vi "Configure Integration.vi"(8 "error in (no error)":errorcluster, 10 "Integration Time (5: 1PLC)":i32(ring)=5 items=["100us", "500us", "1ms", "5ms", "10ms", "1PLC", "100ms", "200ms", "Sample Hold(100 ms)"], 11 "VISA resource name":refnum<visa-resource-name>) -> (0 "error out":errorcluster, 3 "VISA resource name out":refnum<visa-resource-name>)   [LabVIEW 2017, in "ADCMT 6240.lvlib"]
doc: "This VI configures the integration time on the instrument.\n\n<B>Note:</B> Sample Hold can set only at the pulse mode, the pulse-RM mode or the pulse sweep mode."
uses:
  ADCMT 6240.lvlib
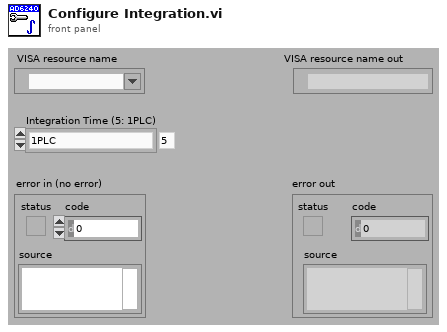
[diagram p1: front panel]
types:
  T1 = typedef "ADCMT 6240.lvlib/Extended User Data.ctl" = cluster{"Trigger Mode":u16, "Output Mode":u16, "Sample Count":i32, "Model":u16}
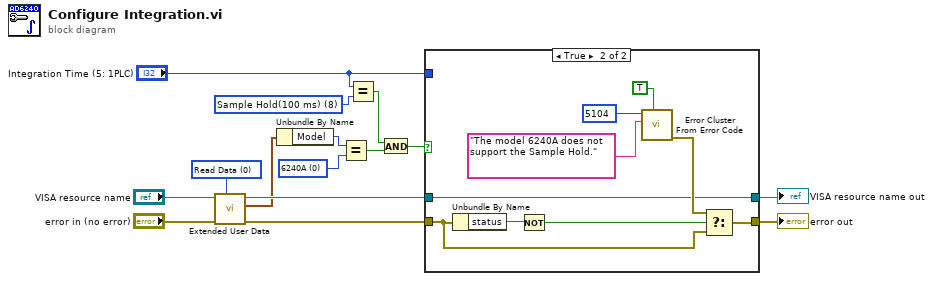
[diagram p0: block diagram]
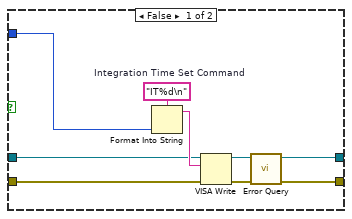
[diagram p2: hidden frame]
diagram:
  w5 = 8 items=["100us", "500us", "1ms", "5ms", "10ms", "1PLC", "100ms", "200ms", "Sample Hold(100 ms)"] ("Integration Time (5: 1PLC)")
  w12 = u16 0 items=["6240A", "6240B"] ("Model")
  w13 = u16 0 items=["Read Data", "Write Data", "Dispose of Data"] ("Action")
  n1 = call "Extended User Data.vi"("Action"=w13, "Error In (no error)"="error in (no error)", "VISA resource name in"="VISA resource name") -> ("Error Out"=w6:errorcluster, "User Data Out"=w7:T1, "VISA resource name out"=w8:refnum<visa-resource-name>)  [unwired: 6 in]
  n2 = Unbundle By Name(w7) -> ("Model"=w11:u16)
  n3 = Equal?(x=w11, y=w12) -> (x = y?=w2:bool)
  n4 = Equal?(x="Integration Time (5: 1PLC)", y=w5) -> (x = y?=w3:bool)
  n5 = And(x=w3, y=w2) -> (x .and. y?=w1:bool)
  n6 = case shown="True" w1 {
    tunnel: [w24 w27] -> w15
    tunnel: [w23 w28] -> w14
    tunnel: w8 -> [w18 w27]
    tunnel: w6 -> [w17 w29]
    tunnel: "Integration Time (5: 1PLC)" -> [w16 _]
    frame False {
      w20 = "IT%d\n"  # Integration Time Set Command
      n7 = Format Into String(format string=w20, w16) -> (resulting string=w19:string)  [unwired: 2 in, 1 out]
      n8 = VISA Write(VISA resource name=w18, write buffer=w19, error in (no error)=w17) -> (VISA resource name out=w21:refnum<visa-resource-name>, error out=w22:errorcluster)  [unwired: 1 out]
      n9 = call "Error Query.vi"("error in (no error)"=w22, "VISA resource name"=w21) -> ("error out"=w23:errorcluster, "VISA resource name out"=w24:refnum<visa-resource-name>)  [unwired: 6 in, 2 out]
    }
    frame True {
      n10 = Unbundle By Name(w29) -> ("status"=w26:bool)
      n11 = Not(x=w26) -> (.not. x?=w31:bool)
      n12 = call <vilib>:"Error Cluster From Error Code.vi"("show call chain? (False)"=TRUE, "error message (\"\")"="The model 6240A does not support the Sample Hold." ("Source (VI Name)"), "error code (0)"=5104 ("Code")) -> ("error out"=w30:errorcluster)  [unwired: 6 in]
      n13 = Select(t=w30, s=w31, f=w29) -> (s? t:f=w28:errorcluster)
    }
  }
  "error out" <- w14
  "VISA resource name out" <- w15
